vi "Get Select Data.vi"(8 "error in":errorcluster) -> (0 "error out":errorcluster, 2 "data out":string[](array[string]))   [LabVIEW 2016]
uses:
  HardWare/Ctrls/HardWare _ Data Queue Manage FGV Operation.ctl
  <vilib>/Analysis/baseanly.llb/Mean (DBL).vi
  MainUI/Config Display Font Size.vi
  <vilib>/Analysis/NI_AALBase.lvlib
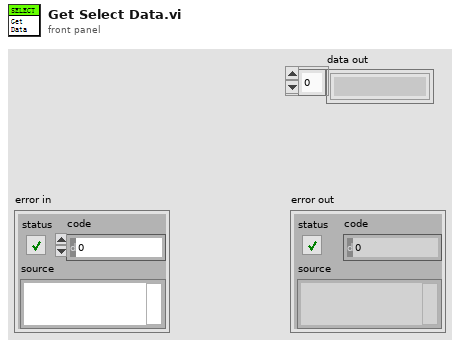
[diagram p1: front panel]
types:
  T1 = typedef "HardWare _ Data Queue Manage FGV Operation.ctl" = enum16{"Initialize", "Add", "Read", "All"}
  T2 = cluster{"Queue Name":string, "ChanTagList[]":string[]}[]
  T3 = cluster{"Channel Font Size":u32, "Channel Value Font Size":u32, "Unit Font Size":u32, "Row Font Size":u32, "Display Precision":u32}
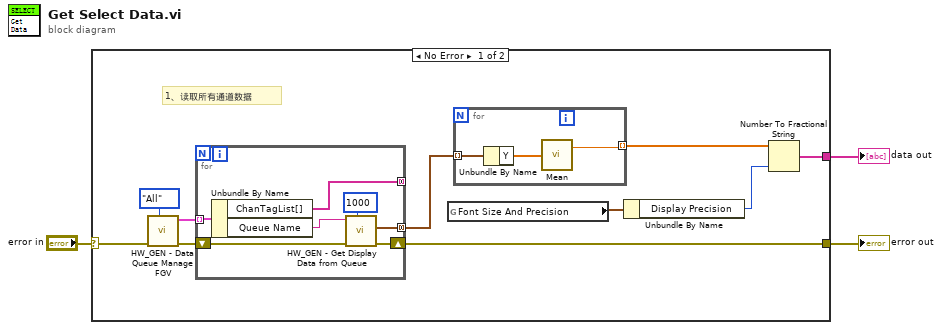
[diagram p0: block diagram]
diagram:
  n1 = case shown="No Error" "error in" {
    selector: "error in" -> [w13 w24]
    tunnel: [w11 w24] -> w2
    tunnel: [w12 _] -> w1
    frame No Error {
      # "1、读取所有通道数据"
      n2 = call "HW_GEN - Data Queue Manage FGV.vi"("Oper."=HardWare___Data_Queue_Manage_FGV_Operation."All", "error in"=w13) -> ("error out"=w8:errorcluster, "AllChanInfo"=w9:T2)  [unwired: 7 in, 1 out]
      n3 = for {
        tunnel: w9 -> [w23] mode=indexing
        shift-right: [w19] -> w11
        shift-left: w8 -> [w21]
        tunnel: [w18] -> w7 mode=concatenating
        tunnel: [w17] -> _ mode=concatenating
        n4 = Unbundle By Name(w23) -> ("ChanTagList[]"=w17:string[], "Queue Name"=w20:string)
        n5 = call "HW_GEN - Get Display Data from Queue.vi"("Time Out(-1)"=1000, "error in"=w21, "Object Name"=w20) -> ("error out"=w19:errorcluster, "data"=w18:waveform(dbl)[])  [unwired: 6 in, 1 out]
      }
      n6 = global read "Config Display Font Size.vi" "Font Size And Precision"() -> (w5:T3)
      n7 = for {
        tunnel: w7 -> [w16] mode=indexing
        tunnel: [w14] -> w4 mode=indexing
        n8 = Unbundle By Name(w16) -> ("Y"=w15:dbl[])
        n9 = call-poly <vilib>:"Mean.vi"("X"=w15) -> ("mean"=w14:dbl)  [unwired: 1 out]
      }
      n10 = Unbundle By Name(w5) -> ("Display Precision"=w6:u32)
      n11 = Number To Fractional String(number=w4, precision (6)=w6) -> (F-format string=w12:string[])  [unwired: 2 in]
    }
    frame Error {
    }
  }
  "error out" <- w2
  "data out" <- w1
